vi "Creators All Created Queues.vi"(9 "Priority?":bool, 10 "Msg Strategy":refnum<class "Msg Strategy.lvclass">, 11 "Hello World Event in":refnum<class "Hello World Event.lvclass">) -> (3 "Hello World Event out":refnum<class "Hello World Event.lvclass">)   [LabVIEW 2021, in "Hello World Event.lvlib" / "Hello World Event.lvclass"]
uses:
  Hello World Event.lvclass
  <vilib>/Nathan Davis/jettl/jettl/Msg Strategy/Msg Strategy.lvclass
  Hello World Event.lvclass/Hello World Event.ctl
  <vilib>/Nathan Davis/jettl/jettl/Event/Event.lvclass
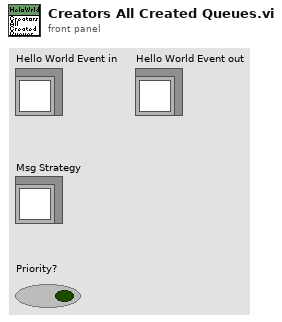
[diagram p1: front panel]
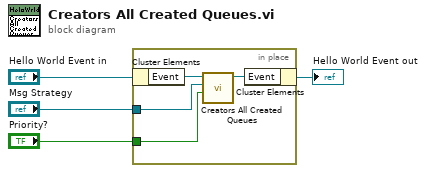
[diagram p0: block diagram]
diagram:
  n1 = in-place {
    in-place-border: "Msg Strategy" -> [w6]
    in-place-border: "Priority?" -> [w5]
    n2 = in-place-cluster #1("Hello World Event in") -> ("Event"=w8:refnum<class "Event.lvclass">)
    n3 = call-dynamic "Creators All Created Queues.vi"("Priority?"=w5, "Msg Strategy"=w6, "Event in"=w8) -> ("Event out"=w7:refnum<class "Event.lvclass">)  [unwired: 8 in]
    n4 = in-place-cluster #1("Event"=w7) -> (→"Hello World Event out":refnum<class "Hello World Event.lvclass">)
  }
